vi "beginFromPreparePass.vi"(9 "begin?":bool, 10 "Game in":refnum<class "Game.lvclass">, 11 "5RobotsNormalGamePlay in":refnum<class "5RobotsNormalGamePlay.lvclass">) -> (2 "Game out":refnum<class "Game.lvclass">, 3 "5RobotsNormalGamePlay out":refnum<class "5RobotsNormalGamePlay.lvclass">)   [LabVIEW 2023, in "5RobotsNormalGamePlay.lvclass"]
uses:
  5RobotsNormalGamePlay.lvclass
  Game_class/Game.lvclass
  Game_class/Game.lvclass/Game.ctl
  Ally_class/Ally.lvclass/Ally.ctl
  5RobotsNormalGamePlay.lvclass/5RobotsNormalGamePlay.ctl
  Playbook_class/Playbook.lvclass/Playbook.ctl
  Write FromPreparePass.vi
  Playbook_class/Read offensive_plays.vi
  Playbook_class/Write offensive_plays.vi
  Game_class/Read OffensiveTeam.vi
  Ally_class/Read DirectOrKickoff.vi
  Ally_class/Ally.lvclass
  Playbook_class/Playbook.lvclass
  Play_class/Play.lvclass
  TestPlay_class/TestPlay.lvclass
  EnemyPossessionAtEnemyFieldPlay_class/EnemyPossessionAtEnemyFieldPlay.lvclass
  EnemyPossessionAtOurFieldPlay_class/EnemyPossessionAtOurFieldPlay.lvclass
  NormalGamePlay_class/NormalGamePlay.lvclass
  IndirectEnemyPlay_class/IndirectEnemyPlay.lvclass
  PrepareKickoffAllyPlay_class/PrepareKickoffAllyPlay.lvclass
  PrepareKickoffEnemyPlay_class/PrepareKickoffEnemyPlay.lvclass
  KickPenaltyAllyPlay_class/KickPenaltyAllyPlay.lvclass
  PreparePenaltyAllyPlay_class/PreparePenaltyAllyPlay.lvclass
  DirectEnemyPlay_class/DirectEnemyPlay.lvclass
  PreparePenaltyEnemyPlay_class/PreparePenaltyEnemyPlay.lvclass
  BallOutOfFieldPlay_class/BallOutOfFieldPlay.lvclass
  StopOffensivePlay_class/StopOffensivePlay.lvclass
  PassPlay_class/PassPlay.lvclass
  DirectKickPlay_class/DirectKickPlay.lvclass
  HaltPlay_class/HaltPlay.lvclass
  PreparePassPlay_class/PreparePassPlay.lvclass
  PassToStriker_class/PassToStriker.lvclass
  PassTo2ndStriker_class/PassTo2ndStriker.lvclass
  SimplePass_class/SimplePass.lvclass
  PrepareRollToPassPlay_class/PrepareRollToPassPlay.lvclass
  PrepareDoublePassPlay_class/PrepareDoublePassPlay.lvclass
  TableWith2ndStrikerPlay_class/TableWith2ndStrikerPlay.lvclass
  TableWithStrikerPlay_class/TableWithStrikerPlay.lvclass
  PrepareTriplePassPlay_class/PrepareTriplePassPlay.lvclass
  ABCPassPlay_class/ABCPassPlay.lvclass
  PreparePassInGame1_class/PreparePassInGame1.lvclass
  ACBPassPlay_class/ACBPassPlay.lvclass
  PrepareKeeperPassPlay_class/PrepareKeeperPassPlay.lvclass
  KeeperPassToStrikerPlay_class/KeeperPassToStrikerPlay.lvclass
  5RobotsPassGamePlay_class/5RobotsPassGamePlay.lvclass
  5RobotsKeeperGame_class/5RobotsKeeperGame.lvclass
  5PreparePassGamePlay_class/5PreparePassGamePlay.lvclass
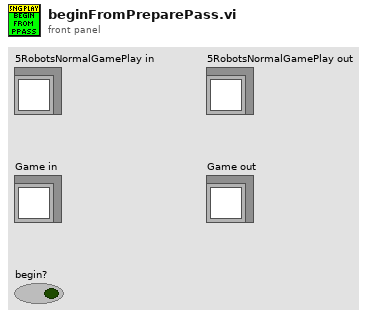
[diagram p1: front panel]
types:
  T1 = typedef "offensive_plays.ctl" = cluster{"Play":refnum<class "Play.lvclass">, "TestPlay":refnum<class "TestPlay.lvclass">, "EnemyPossessionAtEnemyFieldPlay":refnum<class "EnemyPossessionAtEnemyFieldPlay.lvclass">, "EnemyPossessionAtOurFieldPlay":refnum<class "EnemyPossessionAtOurFieldPlay.lvclass">, "NormalGamePlay":refnum<class "NormalGamePlay.lvclass">, "IndirectEnemyPlay":refnum<class "IndirectEnemyPlay.lvclass">, "PrepareKickoffAllyPlay":refnum<class "PrepareKickoffAllyPlay.lvclass">, "PrepareKickoffEnemyPlay":refnum<class "PrepareKickoffEnemyPlay.lvclass">, "KickPenaltyAllyPlay":refnum<class "KickPenaltyAllyPlay.lvclass">, "PreparePenaltyAllyPlay":refnum<class "PreparePenaltyAllyPlay.lvclass">, "DirectEnemyPlay":refnum<class "DirectEnemyPlay.lvclass">, "PreparePenaltyEnemyPlay":refnum<class "PreparePenaltyEnemyPlay.lvclass">, "BallOutOfFieldPlay":refnum<class "BallOutOfFieldPlay.lvclass">, "StopOffensivePlay":refnum<class "StopOffensivePlay.lvclass">, "PassPlay":refnum<class "PassPlay.lvclass">, "DirectKickPlay":refnum<class "DirectKickPlay.lvclass">, "HaltPlay":refnum<class "HaltPlay.lvclass">, "PreparePassPlay":refnum<class "PreparePassPlay.lvclass">, "PassToStrikerPlay":refnum<class "PassToStriker.lvclass">, "PassTo2ndStrikerPlay":refnum<class "PassTo2ndStriker.lvclass">, "SimplePassPlay":refnum<class "SimplePass.lvclass">, "PrepareRollToPassPlay":refnum<class "PrepareRollToPassPlay.lvclass">, "PrepareDoublePassPlay":refnum<class "PrepareDoublePassPlay.lvclass">, "TableWith2ndStrikerPlay":refnum<class "TableWith2ndStrikerPlay.lvclass">, "TableWithStrikerPlay":refnum<class "TableWithStrikerPlay.lvclass">, "PrepareTriplePassPlay":refnum<class "PrepareTriplePassPlay.lvclass">, "ABCPassPlay":refnum<class "ABCPassPlay.lvclass">, "PreparePassInGame1":refnum<class "PreparePassInGame1.lvclass">, "ACBPassPlay":refnum<class "ACBPassPlay.lvclass">, "PrepareKeeperPassPlay":refnum<class "PrepareKeeperPassPlay.lvclass">, "KeeperPassToStrikerPlay":refnum<class "KeeperPassToStrikerPlay.lvclass">, "SimplePass":refnum<class "SimplePass.lvclass">, "SimplePass 2":refnum<class "SimplePass.lvclass">, "5RobotsNormalGamePlay":refnum<class "5RobotsNormalGamePlay.lvclass">, "5RobotsPassGamePlay":refnum<class "5RobotsPassGamePlay.lvclass">, "5RobotsKeeperGame":refnum<class "5RobotsKeeperGame.lvclass">, "5PreparePassGamePlay":refnum<class "5PreparePassGamePlay.lvclass">}
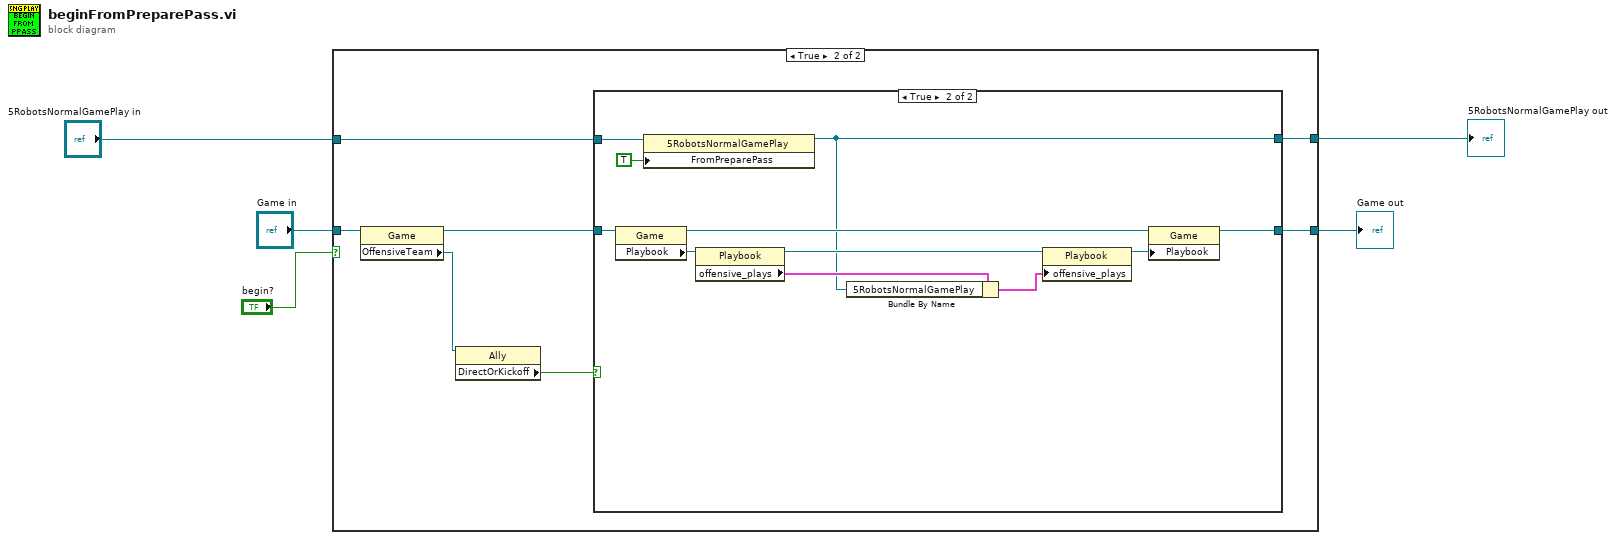
[diagram p0: block diagram]
diagram:
  n1 = case shown="True" "begin?" {
    tunnel: [w7 w12] -> w2
    tunnel: "Game in" -> [w7 w14]
    tunnel: "5RobotsNormalGamePlay in" -> [w6 w10]
    tunnel: [w6 w9] -> w5
    frame False {
    }
    frame True {
      n2 = property class="Game"(reference=w14) -> (reference out=w11:refnum<class "Game.lvclass">, "OffensiveTeam"=w13:refnum<class "Ally.lvclass">)  [unwired: 1 in, 1 out]
      n3 = property class="Ally"(reference=w13) -> ("DirectOrKickoff"=w8:bool)  [unwired: 1 in, 2 out]
      n4 = case shown="True" w8 {
        tunnel: [w16 w24] -> w12
        tunnel: w11 -> [w16 w25]
        tunnel: w10 -> [w15 w26]
        tunnel: [w15 w18] -> w9
        frame False {
        }
        frame True {
          n5 = property class="Game"(reference=w25) -> ("Playbook"=w22:refnum<class "Playbook.lvclass">)  [unwired: 1 in, 2 out]
          n6 = property class="5RobotsNormalGamePlay"(reference=w26, "FromPreparePass"=TRUE) -> (reference out=w18:refnum<class "5RobotsNormalGamePlay.lvclass">)  [unwired: 1 in, 1 out]
          n7 = property class="Playbook"(reference=w22) -> (reference out=w20:refnum<class "Playbook.lvclass">, "offensive_plays"=w21:T1)  [unwired: 1 in, 1 out]
          n8 = Bundle By Name(cluster=w21, "5RobotsNormalGamePlay"=w18) -> (w19:T1)
          n9 = property class="Playbook"(reference=w20, "offensive_plays"=w19) -> (reference out=w23:refnum<class "Playbook.lvclass">)  [unwired: 1 in, 1 out]
          n10 = property class="Game"(reference=w25, "Playbook"=w23) -> (reference out=w24:refnum<class "Game.lvclass">)  [unwired: 1 in, 1 out]
        }
      }
    }
  }
  "5RobotsNormalGamePlay out" <- w5
  "Game out" <- w2
